vi "GetVIsToNotUpdateConnectorPanePatteronOn.vi"(0 "ClassWriterGOOP300 in":refnum<class "ClassWriterGOOP400.lvclass">, 5 "error in (no error)":errorcluster) -> (14 "ClassWriterGOOP300 out":refnum<class "ClassWriterGOOP400.lvclass">, 15 "VIsToNotUpdateConnectorPanePatteronOn":string[](array[string]), 19 "error out":errorcluster)   [LabVIEW 2016, in "ClassWriterGOOP400.lvclass"]
uses:
  <resource>/Framework/Providers/Open_GDS/ClassProviders/Provider_EndevoGOOP400/ClassWriterGOOP400_class/ClassWriterGOOP400.lvclass
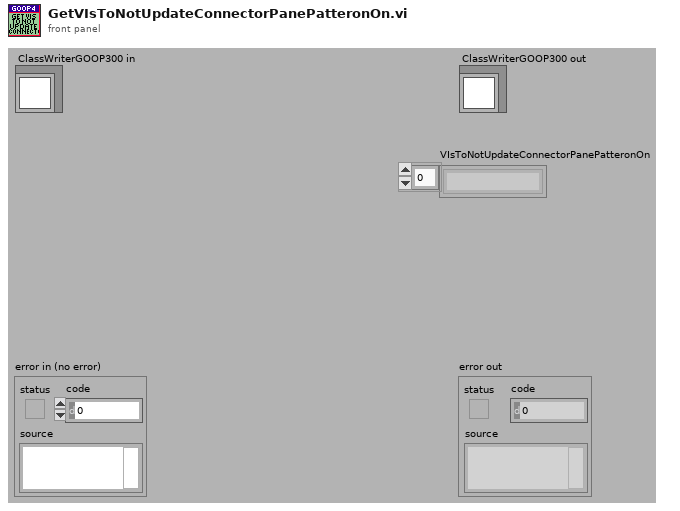
[diagram p1: front panel]
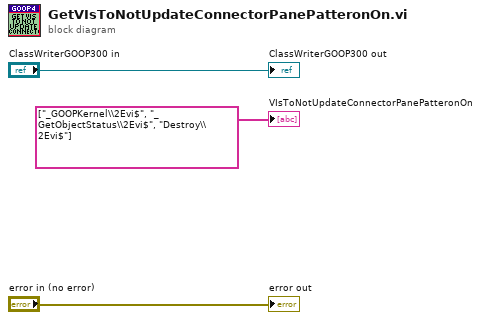
[diagram p0: block diagram]
diagram:
  "ClassWriterGOOP300 out" <- "ClassWriterGOOP300 in"
  "VIsToNotUpdateConnectorPanePatteronOn" <- string[] ["_GOOPKernel\\2Evi$", "_GetObjectStatus\\2Evi$", "Destroy\\2Evi$"] ("VIsToNotUpdateConnectorPanePatteronOn")
  "error out" <- "error in (no error)"
